vi "NEW_Evaluate Loaded Stats.vi"(0 "Stat Array In":string[][](array[string]), 7 "Data Array":string[][](array[string]), 11 "CMDCluster In":T1) -> (4 "Stat Array Out":string[][](array[string]), 15 "Invalid?":bool)   [LabVIEW 2013]
uses:
  TypeDef/Command Cluster.ctl
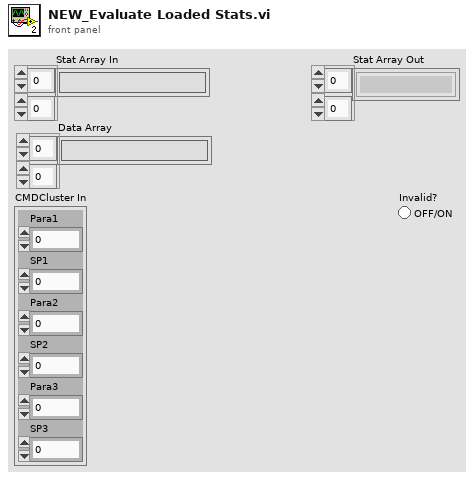
[diagram p1: front panel]
types:
  T1 = typedef "Command Cluster.ctl" = cluster{"Para1":i32, "SP1":dbl, "Para2":i32, "SP2":dbl, "Para3":i32, "SP3":dbl}
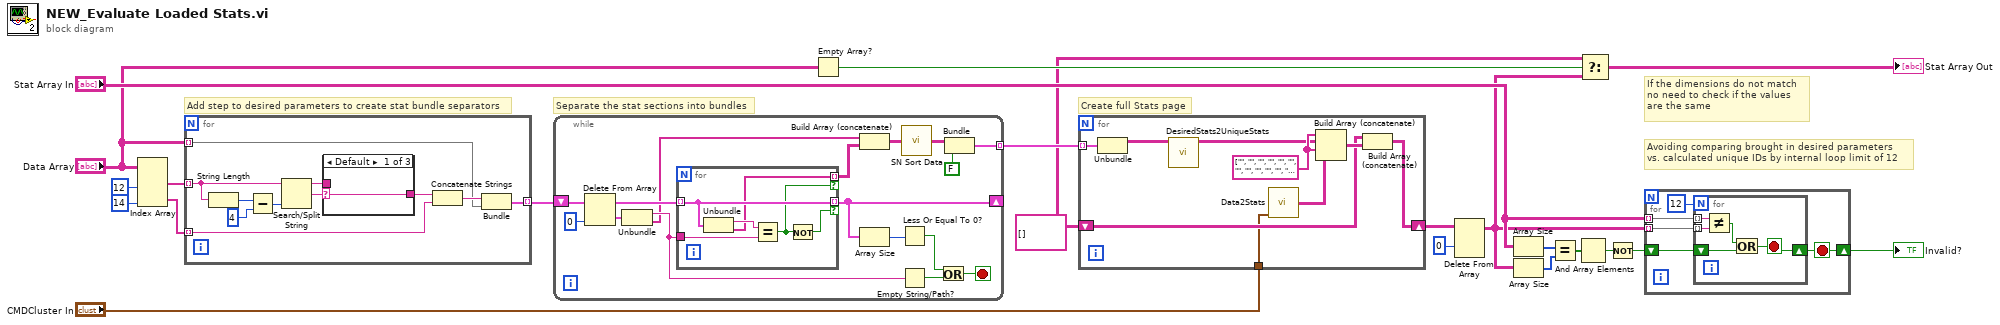
[diagram p0: block diagram]
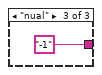
[diagram p3: hidden frame]
diagram:
  w2 = string[][] []
  # "Avoiding comparing brought in desired parameters\nvs. calculated unique IDs by internal loop limit of 12"
  # "Create full Stats page"
  # "If the dimensions do not match\nno need to check if the values\nare the same"
  # "Separate the stat sections into bundles"
  # "Add step to desired parameters to create stat bundle separators"
  n1 = Index Array(array="Data Array", index (col) #1=12 ("disabled index (col)"), index (col) #2=14 ("index (col)")) -> (element #1=w19:string[], element #2=w18:string[])  [unwired: 2 in]
  n2 = for {
    tunnel: w19 -> [w26] mode=indexing
    tunnel: w18 -> [w25] mode=indexing
    tunnel: "Data Array" -> [w23] mode=indexing
    tunnel: [w22] -> w17 mode=indexing
    n3 = String Length(string=w26) -> (length=w27:i32)
    n4 = Subtract(x=w27, y=4) -> (x-y=w30:i32)
    n5 = Search/Split String(string=w26, offset (0)=w30) -> (substring before match=w31:string, match + rest of string=w29:string)  [unwired: 1 in, 1 out]
    n6 = case shown="Default" w29 {
      selector: w29 -> [w33 _ _]
      tunnel: [w33 w34 "-1"] -> w32
      tunnel: w31 -> [_ w34 _]
      frame Default {
      }
      frame " (M)" {
      }
      frame "nual" {
      }
    }
    n7 = Concatenate Strings(w32, w25) -> (w24:string)
    n8 = Bundle(w24, "Data Array"=w23) -> (w22:cluster{string, "Data Array":string[]})  [unwired: 1 in]
  }
  n9 = while {
    shift-right: [w42] -> _
    shift-left: w17 -> [w51]
    tunnel: [w43] -> w16 mode=indexing
    stop <- w39 stop-if-true
    n10 = Delete From Array(array=w51, index=0) -> (deleted portion=w46:cluster{string, "Data Array":string[]}, array with subset deleted=w49:cluster{string, "Data Array":string[]}[])  [unwired: 1 in]
    n11 = Unbundle(w46) -> (w48:string, "Data Array"=w38:string[])
    n12 = for {
      tunnel: w49 -> [w55] mode=indexing
      tunnel: w48 -> [w56]
      tunnel: [w55] -> w42 mode=indexing if=w54
      tunnel: [w52] -> w47 mode=indexing if=w53
      n13 = Unbundle(w55) -> (w57:string, "Data Array"=w52:string[])
      n14 = Equal?(x=w57, y=w56) -> (x = y?=w53:bool)
      n15 = Not(x=w53) -> (.not. x?=w54:bool)
    }
    n16 = Build Array (concatenate)(w38, w47) -> (w37:string[][])
    n17 = Array Size(array=w42) -> (size(s)=w41:i32)
    n18 = Less Or Equal To 0?(x=w41) -> (x <= 0?=w40:bool)
    n19 = Empty String/Path?(string/path=w48) -> (empty?=w45:bool)
    n20 = call "SN Sort Data.vi"("Array In"=w37) -> ("Array Out"=w36:string[][])  [unwired: 14 in]
    n21 = Or(x=w40, y=w45) -> (x .or. y?=w39:bool)
    n22 = Bundle("Array Out"=w36, FALSE) -> (w43:cluster{"Array Out":string[][], bool})  [unwired: 1 in]
  }
  n23 = Empty Array?(array="Data Array") -> (empty?=w4:bool)
  n24 = for {
    tunnel: w16 -> [w66] mode=indexing
    shift-right: [w61] -> w15
    shift-left: w2 -> [w62]
    tunnel: "CMDCluster In" -> [w60]
    w64 = string[] ["", "", "", "", "", "", "", "", "", "", "", "", "", ""]
    n25 = Unbundle(w66) -> ("Array Out"=w59:string[][])  [unwired: 1 out]
    n26 = call "DesiredStats2UniqueStats.vi"("StatCluster In"=w59) -> ("StatCluster Out"=w58:string[][])  [unwired: 10 in]
    n27 = call "Data2Stats.vi"("CMDCluster In"=w60) -> ("StatsOut"=w65:string[][])  [unwired: 14 in]
    n28 = Build Array (concatenate)(w64, w58, w64, w65) -> (w63:string[][])
    n29 = Build Array (concatenate)(w62, w63) -> (w61:string[][])
  }
  n30 = Delete From Array(array=w15, index (row)=0) -> (array with subset deleted=w3:string[][])  [unwired: 2 in, 1 out]
  n31 = Array Size(array="Stat Array In") -> (size(s)=w9:i32[])
  n32 = Array Size(array=w3) -> (size(s)=w10:i32[])
  n33 = Equal?(x=w9, y=w10) -> (x = y?=w11:bool[])
  n34 = And Array Elements(Boolean array=w11) -> (logical AND=w12:bool)
  n35 = Select(t=w2, s=w4, f=w3) -> (s? t:f=→"Stat Array Out":string[][])
  n36 = Not(x=w12) -> (.not. x?=w7:bool)
  n37 = for {
    tunnel: "Stat Array In" -> [w71] mode=indexing
    tunnel: w3 -> [w70] mode=indexing
    shift-right: [w68] -> w13
    shift-left: w7 -> [w69]
    stop <- w68 stop-if-true
    n38 = for {
      N: 12 -> [_]
      tunnel: w71 -> [w76] mode=indexing
      tunnel: w70 -> [w75] mode=indexing
      shift-right: [w72] -> w68
      shift-left: w69 -> [w74]
      stop <- w72 stop-if-true
      n39 = Not Equal?(x=w76, y=w75) -> (x != y?=w73:bool)
      n40 = Or(x=w73, y=w74) -> (x .or. y?=w72:bool)
    }
  }
  "Invalid?" <- w13
